vi "Setup.vi"(11 "Dev Panel in":refnum<class "Dev Panel.lvclass">) -> (0 "error out":errorcluster, 3 "Dev Panel out":refnum<class "Dev Panel.lvclass">)   [LabVIEW 2021, in "Dev Panel.lvclass"]
uses:
  Dev Panel.lvclass
  Dev Panel.lvclass/Dev Panel.ctl
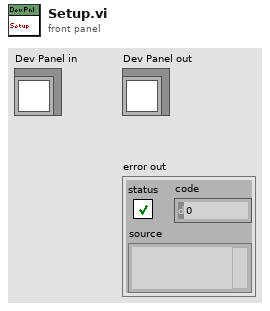
[diagram p1: front panel]
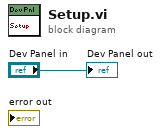
[diagram p0: block diagram]
diagram:
  "Dev Panel out" <- "Dev Panel in"
